vi "Experiment_treatment1_ArtemVer1KG.vi"() -> ()   [LabVIEW 2018]
uses:
  <vilib>/Analysis/1siggen.llb/Ramp Pattern by Samples.vi
  <vilib>/Utility/file.llb/Read From Spreadsheet File (DBL).vi
  <vilib>/Analysis/NI_AALBase.lvlib
  cluster_ip_dll/x64/Release/cluster_ip.dll
panel:
  in  "ratio_perm":dbl=1.0
  in  "length":i32=199847
  out "size(s)":i32[](array[numeric])=[199847, 4]
  out "Working time":dbl=10.736
  in  "Array":string[](array[string])=["Number", "MSE", "Eff. Deg. of Freedom", "Conf. interval size", "Nearest param 1", "Nearest param 2", "Nearest param 3", "Nearest param 4", "Math Exp of param 1", "Math Exp of param 2", "Math Exp of param 3", "Math Exp of param 4", "Stand Dev of param 1", "Stand Dev of param 2", "Stand Dev of param 3", "Stand Dev of param 4", "HPD Intercepts"]
  out "Clusters":i32=2296
  out "Tree built":i32=1
  out "k":dbl=5.363132492919857
  out "Stand Dev":dbl[](array[numeric])=[0.14074417999043268, 0.054181492882835885, 0.0033921981697429128, 12.524756434619329]
  out "Math Exp":dbl[](array[numeric])=[0.6707029123050608, 0.14943200368425694, 1.3769697677746422, 21.22968016405946]
  in  "Database type":u16(ring) items=["Random", "Regular", "Piecewise regular", "DiRect (not realized)"]
  out "MSE":dbl
  out "Nearest Params":sgl[](array[numeric])=[0.68445736, 0.106504805, 1.3702419, 48.924232]
  in  "Load":bool=TRUE
  in  "Params bounds":sgl[][](array[numeric])=[[0.5, 2.12], [0.1, 1.0], [1.37, 1.39], [0.0, 90.0]]
  in  "Database path":path=path "E:/OnEngFiles - science/test labview/4_add_cluster_lib/Plt_200k_h.db"
  in  "Angle bounds":i32[](array[numeric])=[10, 70]
  in  "Path to indicatrices":path=path "E:/OnEngFiles - science/test labview/4_add_cluster_lib/experiment_1000.txt"
  in  "How many to process":u16(ring)=100 items=["All (889)"=889, "100"=100, "300"=300, "1000"=1000]
  in  "Launch":bool=TRUE
  in  "Tab Control":enum32{"Nearest Indicatrix"}(tab)
  out "XY Graph":cluster{"Y":dbl[], "Y":dbl[]}[](graph)=[{"Y"=[10.0, 11.0, 12.0, 13.0, 14.0, 15.0, 16.0, 17.0, 18.0, 19.0, 20.0, 21.0, 22.0, 23.0, 24.0, 25.0, 26.0, 27.0, 28.0, 29.0, 30.0, 31.0, 32.0, 33.0, 34.0, 35.0, 36.0, 37.0, 38.0, 39.0, 40.0, 41.0, 42.0, 43.0, 44.0, 45.0, 46.0, 47.0, 48.0, 49.0, 50.0, 51.0, 52.0, 53.0, 54.0, 55.0, 56.0, 57.0, 58.0, 59.0, 60.0], "Y"=[3.584928234374043e-05, 6.087175402032172e-05, 9.562049901976253e-05, 0.00014104691333700342, 0.00019757729815979622, 0.0002651135616544077, 0.00034308135664397625, 0.0004305081801215161, 0.0005261160539134097, 0.0006284168548823555, 0.0007358019994202503, 0.0008466213987461039, 0.000959249146877231, 0.001072135255465285, 0.0011838439896287526, 0.0012930801075181364, 0.0013987046879531642, 0.0014997423548416817, 0.0015953816629734523, 0.0016849702645666232, 0.0017680062781895245, 0.0018441270646478013, 0.0019130963996333134, 0.0019747908332749266, 0.0020291858490397796, 0.0020763422814356666, 0.0021163933237562708, 0.002149532352204729, 0.0021760017087887502, 0.0021960825196998424, 0.0022100855757161406, 0.0022183432638865374, 0.002221202512987111, 0.002219018696900437, 0.002212150428362565, 0.0022009551689452394, 0.0021857855784477988, 0.002166986527051351, 0.0021448926958249283, 0.0021198266948269017, 0.002092097632614167, 0.00206200007607233, 0.0020298133448228444, 0.001995801089834237, 0.001960211111111111, 0.0019232753743506287, 0.001885210191172391, 0.0018462165319028346, 0.001806480443909125, 0.0017661735521253483, 0.0017254536217018342]}, {"Y"=[10.0, 11.0, 12.0, 13.0, 14.0, 15.0, 16.0, 17.0, 18.0, 19.0, 20.0, 21.0, 22.0, 23.0, 24.0, 25.0, 26.0, 27.0, 28.0, 29.0, 30.0, 31.0, 32.0, 33.0, 34.0, 35.0, 36.0, 37.0, 38.0, 39.0, 40.0, 41.0, 42.0, 43.0, 44.0, 45.0, 46.0, 47.0, 48.0, 49.0, 50.0, 51.0, 52.0, 53.0, 54.0, 55.0, 56.0, 57.0, 58.0, 59.0, 60.0], "Y"=[0.0032144944874749623, 0.0032132298573099827, 0.0029659495363371217, 0.002712444976221678, 0.0026041146328709443, 0.0026259121642624654, 0.002644837766779372, 0.00252843040674818, 0.002242430201747389, 0.0018692780710884763, 0.0015507701572525703, 0.0014033129107546734, 0.0014598002632086123, 0.0016651567756611541, 0.0019170085087040311, 0.0021208737801508017, 0.0022290668182410028, 0.002248300373317722, 0.00222018160530276, 0.00219078906764674, 0.00218647057471567, 0.002205583659012032, 0.0022259928432159367, 0.002220926031811844, 0.00217379465770865, 0.0020852619171353236, 0.001970885484555106, 0.001852323331685977, 0.0017474430288977488, 0.0016641427256584055, 0.0016000347051028934, 0.0015469366635793708, 0.0014969545376869507, 0.0014467263688878807, 0.0013979689937462982, 0.0013547633161661095, 0.0013197453682908813, 0.0012916557375020025, 0.0012655875700386733, 0.0012355249800443844, 0.0011974685704525838, 0.0011512530107925744, 0.0011000865603667544, 0.0010482239528080827, 0.0009982067125814931, 0.0009492368672763391, 0.0008975231352131822, 0.0008383424657175091, 0.0007687260034128252, 0.0006895054184360893, 0.0006059307798655672]}]
  in  "Show graphs":bool
  in  "Calc ME and SD":bool=TRUE
  in  "Clusterization":bool=TRUE
  in  "Use saved tree":bool
  in  "Database path 2":path=path "E:/OnEngFiles - science/test labview/4_add_cluster_lib/complite program/Experiment_treatment1_ArtemVer5_KG02/test_data"
  out "Progress bar":u8(slide)=100 scale=0.0..100.0
  in  "output cluster":T1
  # "Database setup"
  # "Experiment setup"
  # "±"
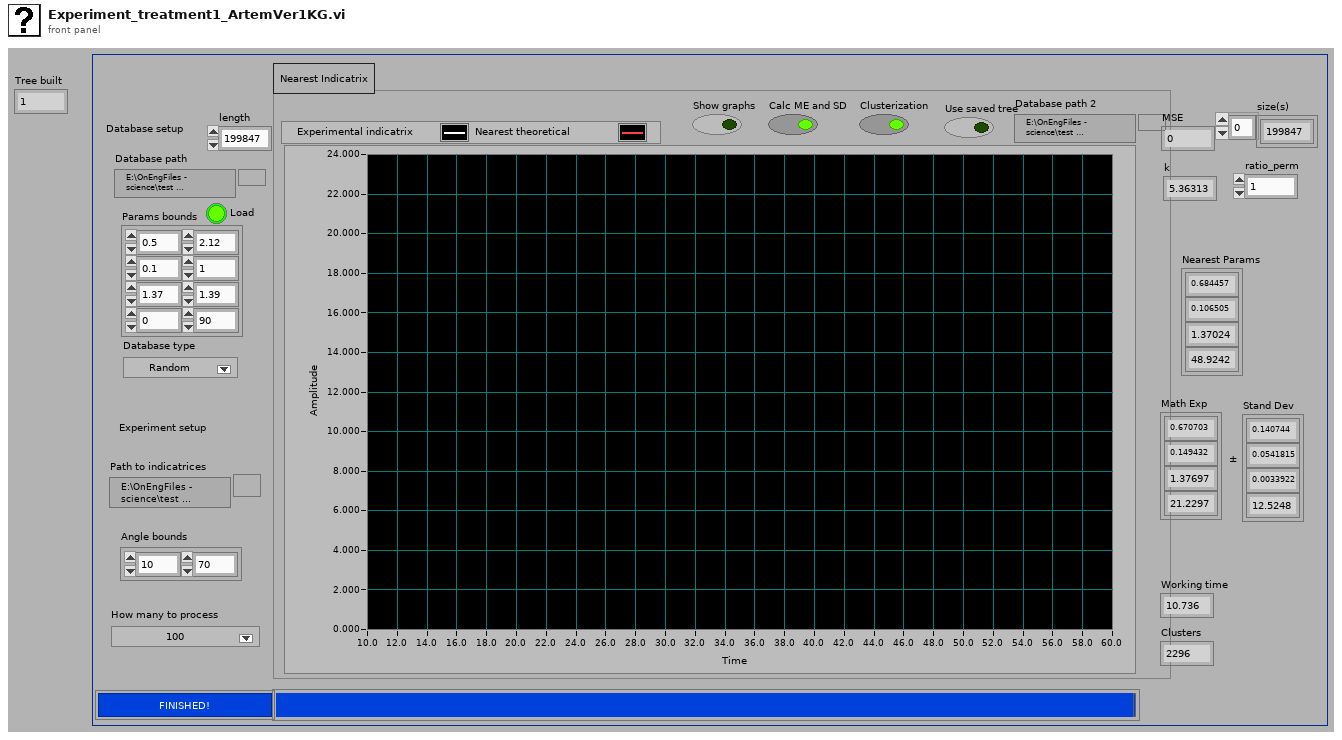
[diagram p1: front panel]
types:
  T1 = cluster{"Angles start":dbl, "Angles end":dbl, "Number of angles":i32, "Params bounds":sgl[][], "Params":sgl[][], "Indicatrices":sgl[][]}
  T2 = typedef "LVStringsAndValuesArrayTypeDef_U16.ctl" = cluster{"String":string, "Value":u16}[]
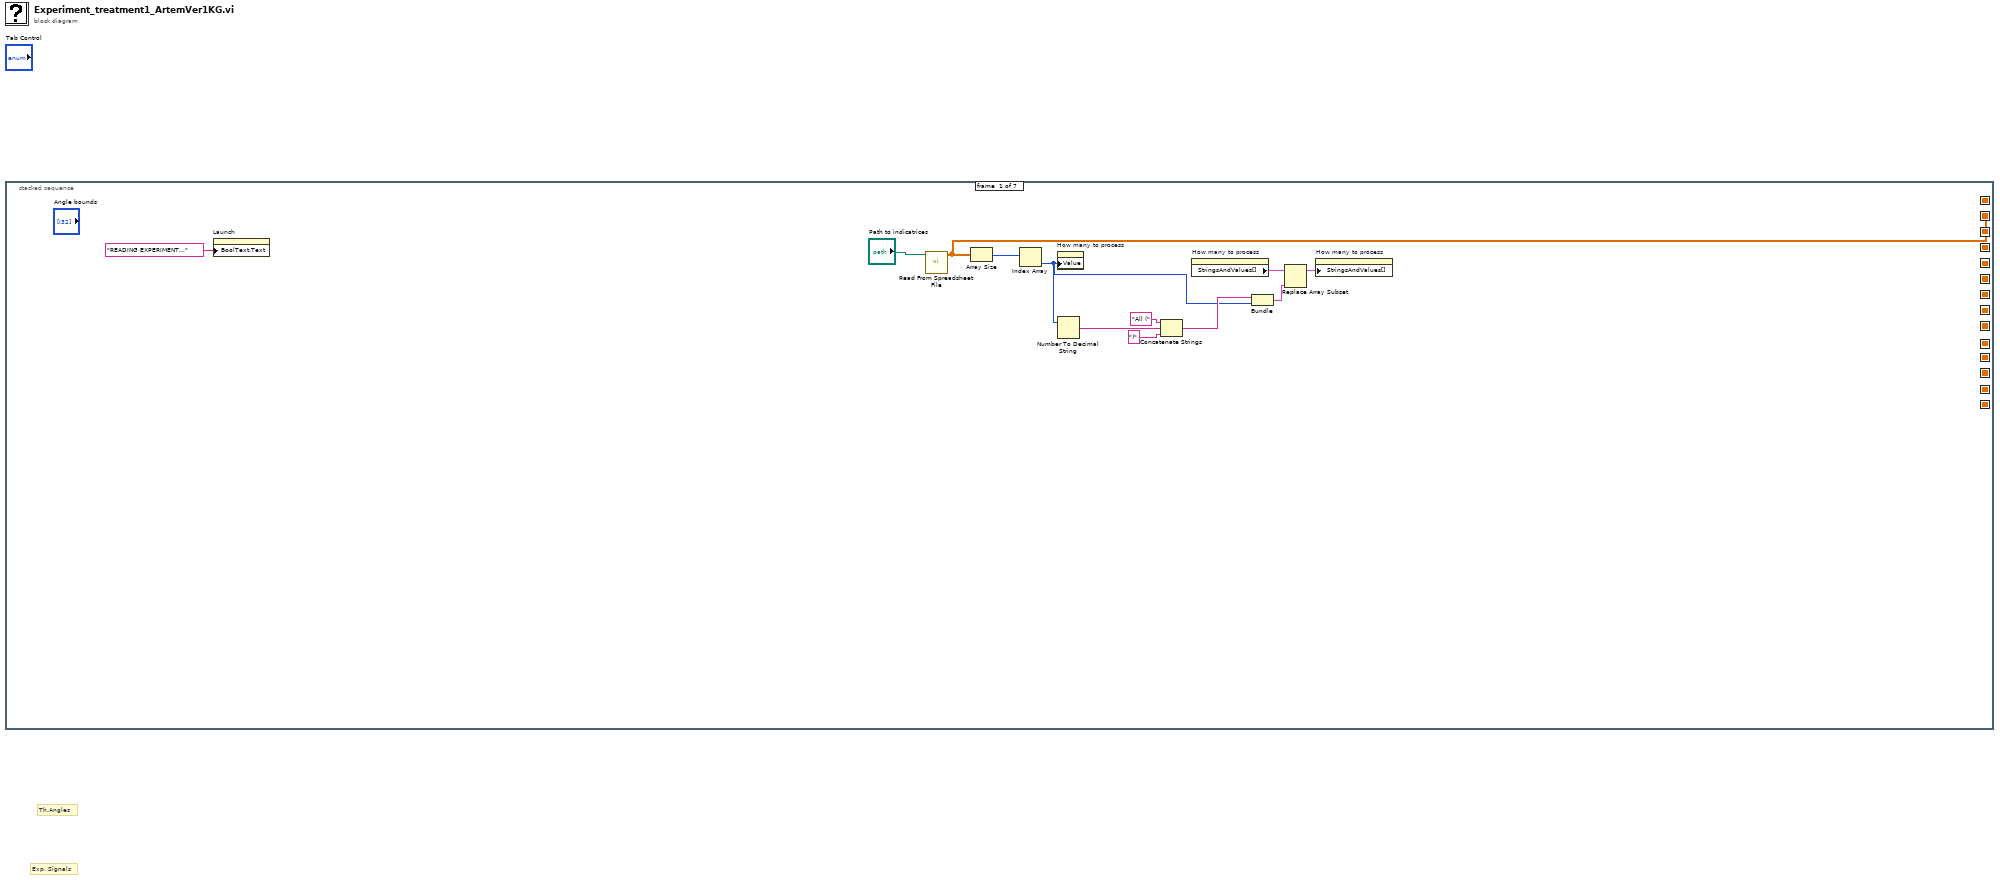
[diagram p0: block diagram]
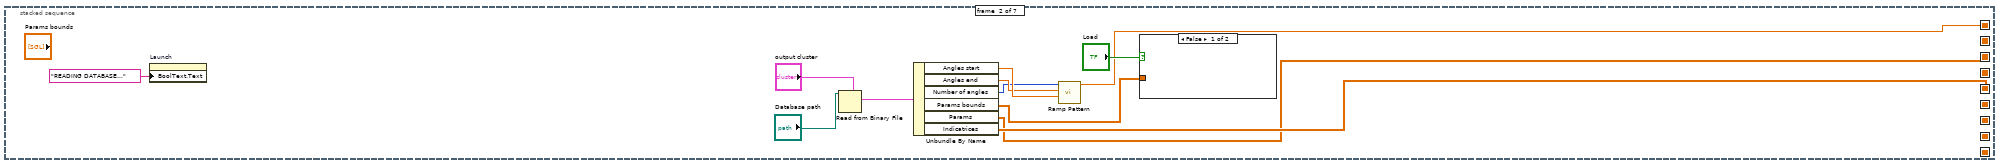
[diagram p2: hidden frame]
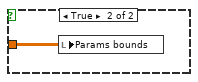
[diagram p3: hidden frame]
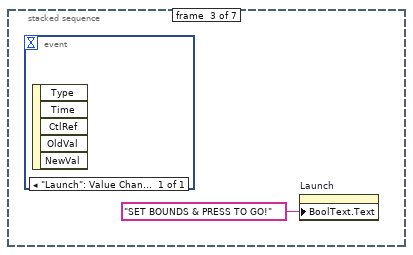
[diagram p4: hidden frame]
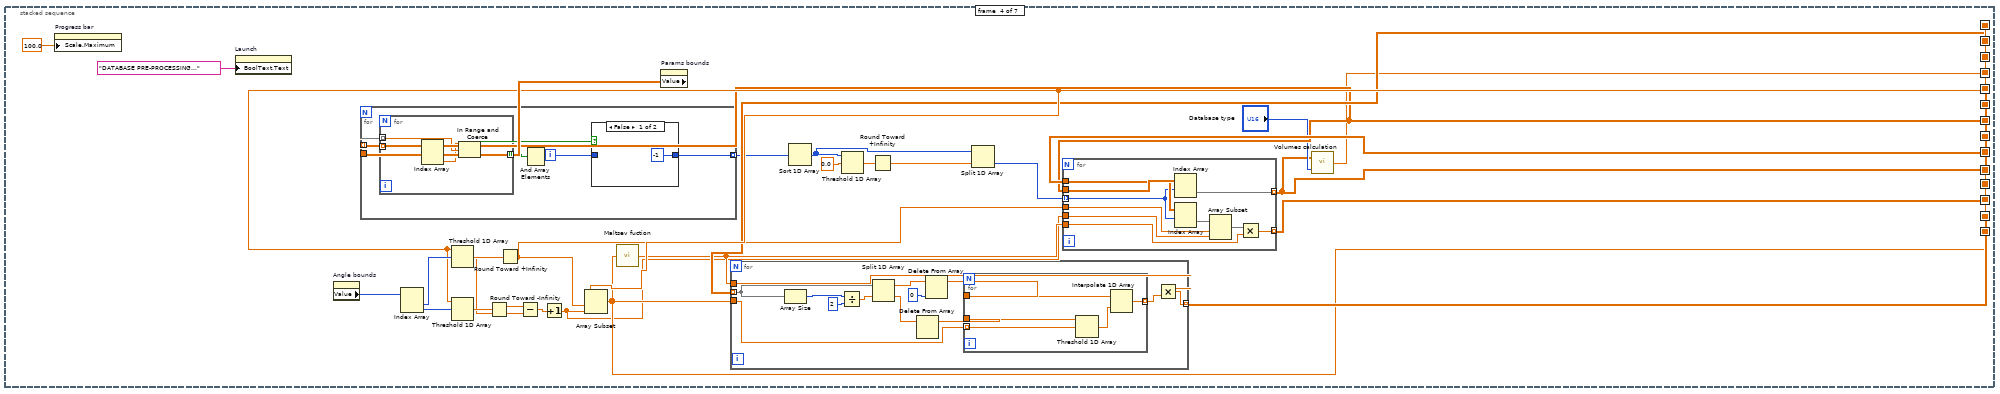
[diagram p5: hidden frame]
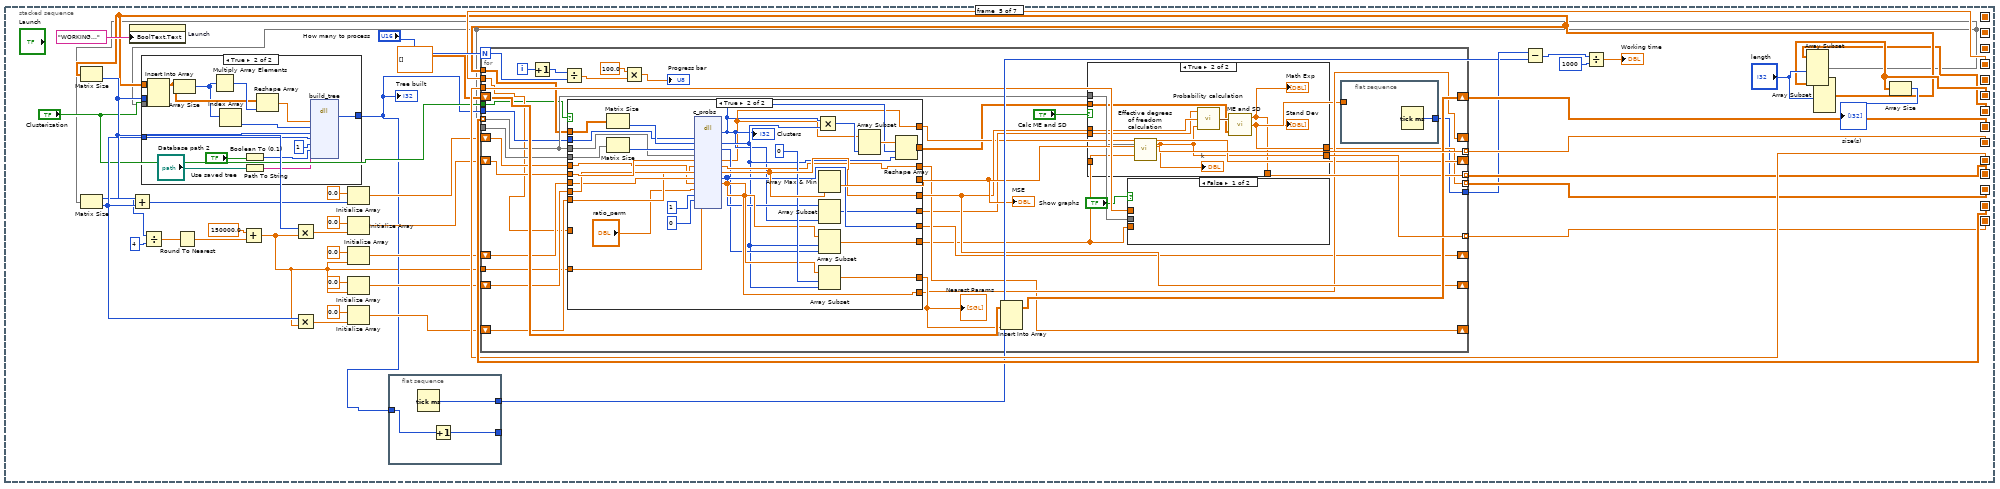
[diagram p7: hidden frame]
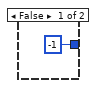
[diagram p8: hidden frame]
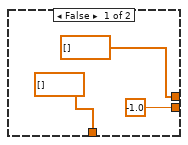
[diagram p9: hidden frame]
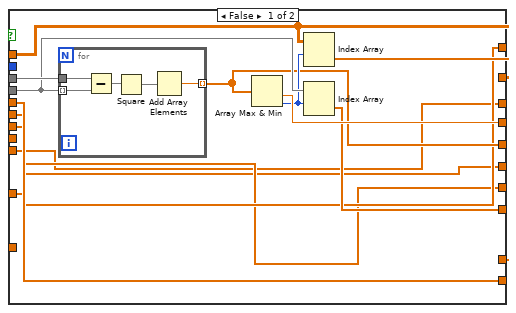
[diagram p10: hidden frame]
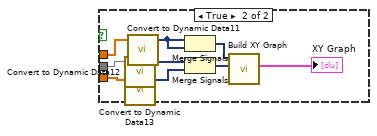
[diagram p11: hidden frame]
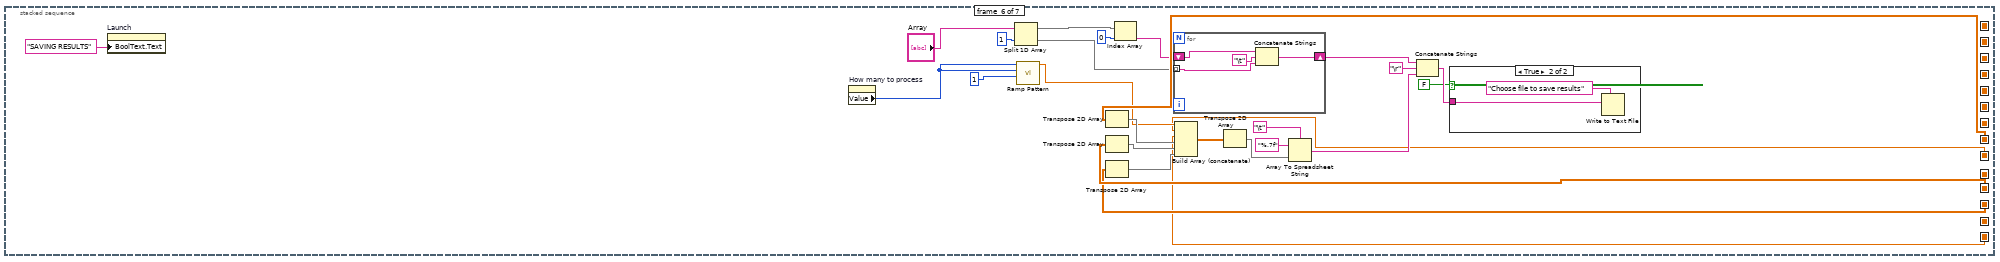
[diagram p12: hidden frame]
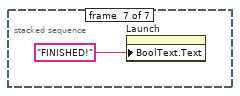
[diagram p14: hidden frame]
diagram:
  # "Th.Angles"
  # "Exp. Signals"
  n1 = stacked-sequence {
    seq-local: [_ w14 _ _ _ _ _] -> [_ _ _ w30 _ _ _]
    seq-local: [_ w21 _ _ _ _ _] -> [_ _ _ w42 _ _ _]
    seq-local: [w1 _ _ _ _ _ _] -> [_ _ _ w45 _ _ _]
    seq-local: [_ w19 _ _ _ _ _] -> [_ _ _ w49 _ _ _]
    seq-local: [_ _ _ w27 _ _ _] -> [_ _ _ _ w101 _ _]
    seq-local: [_ _ _ w41 _ _ _] -> [_ _ _ _ w99 _ _]
    seq-local: [_ _ _ w44 _ _ _] -> [_ _ _ _ w139 _ _]
    seq-local: [_ _ _ w43 _ _ _] -> [_ _ _ _ w138 _ _]
    seq-local: [_ _ _ w29 _ _ _] -> [_ _ _ _ w136 _ _]
    seq-local: [_ _ _ _ w134 _ _] -> [_ _ _ _ _ w293 _]
    seq-local: [_ _ _ _ w135 _ _] -> [_ _ _ _ _ w278 _]
    seq-local: [_ _ _ _ w133 _ _] -> [_ _ _ _ _ w292 _]
    seq-local: [_ _ _ _ w132 _ _] -> [_ _ _ _ _ w291 _]
    seq-local: [_ _ _ _ w131 _ _] -> [_ _ _ _ _ w276 _]
    frame #0 {
      n2 = property on="Launch" class="Bool (strict)"("BoolText.Text"="READING EXPERIMENT..." ("Boolean Text.Text")) -> ()  [unwired: 2 in, 2 out]
      n3 = call-poly <vilib>:"Read From Spreadsheet File.vi"("file path (dialog if empty)"="Path to indicatrices") -> ("all rows"=w1:dbl[][])  [unwired: 6 in, 4 out]
      n4 = Array Size(array=w1) -> (size(s)=w6:i32[])
      n5 = Index Array(array=w6) -> (element=w2:i32)  [unwired: 1 in]
      n6 = property on="How many to process" class="Ring (strict)"("Value"=w2) -> ()  [unwired: 2 in, 2 out]
      n7 = Number To Decimal String(number=w2) -> (decimal integer string=w3:string)  [unwired: 1 in]
      n8 = Concatenate Strings("All (" ("String"), w3, ")" ("String")) -> (w5:string)
      n9 = property on="How many to process" class="Ring (strict)"() -> ("StringsAndValues[]"=w10:T2)  [unwired: 2 in, 2 out]
      n10 = Bundle(w5, w2) -> (w8:cluster{string, i32})  [unwired: 1 in]
      n11 = Replace Array Subset(array=w10, new element=w8) -> (w11:T2)  [unwired: 1 in]
      n12 = property on="How many to process" class="Ring (strict)"("StringsAndValues[]"=w11) -> ()  [unwired: 2 in, 2 out]
    }
    frame #1 {
      n13 = property on="Launch" class="Bool (strict)"("BoolText.Text"="READING DATABASE..." ("Boolean Text.Text")) -> ()  [unwired: 2 in, 2 out]
      n14 = Read from Binary File(5:"output cluster", 11:"Database path") -> (2:w24:T1)  [unwired: 4 in, 3 out]
      n15 = Unbundle By Name(w24) -> ("Angles start"=w20:dbl, "Angles end"=w18:dbl, "Number of angles"=w17:i32, "Params bounds"=w16:sgl[][], "Params"=w14:sgl[][], "Indicatrices"=w21:sgl[][])
      n16 = call-poly <vilib>:"Ramp Pattern.vi"("start"=w20, "end"=w18, "samples"=w17) -> ("Ramp Pattern"=w19:dbl[])  [unwired: 7 in, 1 out]
      n17 = case shown="False" "Load" {
        tunnel: w16 -> [_ w25]
        frame False {
        }
        frame True {
          n18 = local write "Params bounds"(w25) -> ()
        }
      }
    }
    frame #2 {
      n19 = event shown="[0] \"Launch\": Value Change" {
        selector: _ -> [_]
        dyn-events: _ -> [_]
        timeout: _ -> [_]
        event "Launch": Value Change {
          n20 = event-data() -> ()  [unwired: 1 in, 5 out]
        }
      }
      n21 = property on="Launch" class="Bool (strict)"("BoolText.Text"="SET BOUNDS & PRESS TO GO!" ("Boolean Text.Text")) -> ()  [unwired: 2 in, 2 out]
    }
    frame #3 {
      n22 = property on="Progress bar" class="Slide (strict)"("Scale.Maximum"=100.0 ("Scale.Range:Maximum")) -> ()  [unwired: 2 in, 2 out]
      n23 = property on="Launch" class="Bool (strict)"("BoolText.Text"="DATABASE PRE-PROCESSING..." ("Boolean Text.Text")) -> ()  [unwired: 2 in, 2 out]
      n24 = property on="Angle bounds" class="Arr (strict)"() -> ("Value"=w53:i32[])  [unwired: 2 in, 2 out]
      n25 = Index Array(array=w53) -> (element #1=w52:i32, element #2=w46:i32)  [unwired: 2 in]
      n26 = Threshold 1D Array(2:w52, 3:w49) -> (0:w51:dbl)  [unwired: 1 in]
      n27 = Threshold 1D Array(2:w46, 3:w49) -> (0:w50:dbl)  [unwired: 1 in]
      n28 = Round Toward -Infinity(1:w50) -> (0:w48:dbl)
      n29 = Round Toward +Infinity(x=w51) -> (ceil(x): smallest int >= x=w38:dbl)
      n30 = Subtract(x=w48, y=w38) -> (x-y=w47:dbl)
      n31 = Increment(x=w47) -> (x+1=w39:dbl)
      n32 = Array Subset(array=w49, index=w38, length=w39) -> (w43:dbl[])
      n33 = call "Maltsev fuction.vi"("Angles"=w43) -> ("Maltsev fuction"=w40:dbl[])
      n34 = property on="Params bounds" class="Arr (strict)"() -> ("Value"=w54:sgl[][])  [unwired: 2 in, 2 out]
      n35 = for {
        tunnel: w30 -> [w87] mode=indexing
        tunnel: w54 -> [w89]
        tunnel: [w84] -> w37 mode=indexing
        i -> [w85]
        n36 = for {
          tunnel: w89 -> [w96] mode=indexing
          tunnel: w87 -> [w95] mode=indexing
          tunnel: [w92] -> w88 mode=indexing
          n37 = Index Array(array=w96) -> (element #1=w94:sgl, element #2=w93:sgl)  [unwired: 2 in]
          n38 = In Range and Coerce(upper limit=w93, x=w95, lower limit=w94) -> (In Range?=w92:bool)  [unwired: 1 out]
        }
        n39 = And Array Elements(Boolean array=w88) -> (logical AND=w86:bool)
        n40 = case shown="False" w86 {
          tunnel: w85 -> [_ w91]
          tunnel: [-1 w91] -> w84
          frame False {
          }
          frame True {
          }
        }
      }
      n41 = for {
        tunnel: w45 -> [w72] mode=indexing
        tunnel: w43 -> [w69]
        tunnel: w40 -> [w68]
        tunnel: [w66] -> w44 mode=indexing
        n42 = Array Size(array=w72) -> (size(s)=w76:i32)
        n43 = Divide(x=w76, y=2) -> (x/y=w75:dbl)
        n44 = Split 1D Array(array=w72, index=w75) -> (first subarray=w78:dbl[], second subarray=w77:dbl[])
        n45 = Delete From Array(array=w77) -> (array with subset deleted=w70:dbl[])  [unwired: 2 in, 1 out]
        n46 = Delete From Array(array=w78, index=0) -> (array with subset deleted=w71:dbl[])  [unwired: 1 in, 1 out]
        n47 = for {
          tunnel: w71 -> [w82]
          tunnel: w70 -> [w81]
          tunnel: w69 -> [w80] mode=indexing
          tunnel: [w79] -> w67 mode=indexing
          n48 = Threshold 1D Array(2:w80, 3:w81) -> (0:w83:dbl)  [unwired: 1 in]
          n49 = Interpolate 1D Array(1:w83, 2:w82) -> (0:w79:dbl)
        }
        n50 = Multiply(x=w68, y=w67) -> (x*y=w66:dbl[])
      }
      n51 = Sort 1D Array(array=w37) -> (sorted array=w33:i32[])
      n52 = Threshold 1D Array(2:0.0 ("threshold y"), 3:w33) -> (0:w35:dbl)  [unwired: 1 in]
      n53 = Round Toward +Infinity(x=w35) -> (ceil(x): smallest int >= x=w34:dbl)
      n54 = Split 1D Array(array=w33, index=w34) -> (second subarray=w32:i32[])  [unwired: 1 out]
      n55 = for {
        tunnel: w30 -> [w65]
        tunnel: w42 -> [w64]
        tunnel: [w63] -> w27 mode=indexing
        tunnel: [w60] -> w41 mode=indexing
        tunnel: w40 -> [w59]
        tunnel: w39 -> [w58]
        tunnel: w38 -> [w57]
        tunnel: w32 -> [w56] mode=indexing
        n56 = Index Array(array=w65, index (row)=w56) -> (element=w63:sgl[])  [unwired: 1 in]
        n57 = Index Array(array=w64, index (row)=w56) -> (element=w61:sgl[])  [unwired: 1 in]
        n58 = Array Subset(array=w61, index=w57, length=w58) -> (w62:sgl[])
        n59 = Multiply(x=w62, y=w59) -> (x*y=w60:dbl[])
      }
      n60 = call "Volumes calculation.vi"("Ring"="Database type", "Params"=w27) -> ("Volumes"=w29:sgl[])
    }
    frame #4 {
      n61 = property on="Launch" class="Bool (strict)"("BoolText.Text"="WORKING..." ("Boolean Text.Text")) -> ()  [unwired: 2 in, 2 out]
      n62 = flat-sequence {
        tunnel: [w144] -> w109
        tunnel: w104 -> [w143]
        tunnel: [w142] -> _
        frame #0 {
          n63 = Tick Count (ms)() -> (millisecond timer value=w144:u32)
          n64 = Increment(x=w143) -> (x+1=w142:i32)
        }
      }
      n65 = Array Subset(array=w99, length (row)="length") -> (w98:dbl[][])  [unwired: 3 in]
      n66 = Matrix Size(0:w98) -> (1:w114:i32, 2:w117:i32)
      n67 = Divide(x=w114, y=4) -> (x/y=w112:dbl)
      n68 = Round To Nearest(number=w112) -> (nearest integer value=w111:dbl)
      n69 = Add(x=150000.0 ("element"), y=w111) -> (x+y=w97:dbl)
      n70 = Multiply(x=w117, y=w97) -> (x*y=w118:dbl)
      n71 = Initialize Array(0.0 ("element"), w97) -> (w121:dbl[])
      n72 = Initialize Array(0.0 ("element"), w97) -> (w122:dbl[])
      n73 = Initialize Array(0.0 ("element"), w118) -> (w116:dbl[])
      n74 = Array Subset(array=w101, length (row)="length") -> (w100:sgl[][])  [unwired: 3 in]
      n75 = Matrix Size(0:w100) -> (2:w130:i32)  [unwired: 1 out]
      n76 = Add(x=w130, y=w117) -> (x+y=w129:i32)
      n77 = case shown="True" "Clusterization" {
        tunnel: w130 -> [_ w160]
        tunnel: w100 -> [_ w153]
        tunnel: w98 -> [_ w152]
        tunnel: [-1 ("return type") w151] -> w104
        tunnel: w117 -> [_ w150]
        frame False {
        }
        frame True {
          n78 = Insert Into Array(array=w153, index (col)=w160, new element=w152) -> (w155:sgl[][])  [unwired: 1 in]
          n79 = Array Size(array=w155) -> (size(s)=w154:i32[])
          n80 = Multiply Array Elements(1:w154) -> (0:w156:i32)
          n81 = Index Array(array=w154) -> (element=w158:i32)  [unwired: 1 in]
          n82 = Path To String(path="Database path 2") -> (string=w146:string)
          n83 = Boolean To (0,1)(Boolean="Use saved tree") -> (0, 1=w148:i16)
          n84 = Reshape Array(w155, w156) -> (w157:sgl[])
          n85 = dll-call lib="E:/OnEngFiles - science/test labview/4_add_cluster_lib/git_version/Cluster_IP/actual_code/cluster_ip_dll/x64/Release/cluster_ip.dll" fn="build_tree"("data"=w157, "number_points"=w158, "hiden_size"=w160, "mesured_size"=w150, "save"=1, "use_saved"=w148, "folder_name"=w146) -> ("return type"=w151:i32)  [unwired: 10 in, 2 out]
        }
      }
      "Tree built" <- w104
      n86 = Multiply(x=w130, y=w97) -> (x*y=w128:dbl)
      n87 = Initialize Array(0.0 ("element"), w129) -> (w120:dbl[])
      n88 = Initialize Array(0.0 ("element"), w128) -> (w123:dbl[])
      n89 = for {
        N: "How many to process" -> [w195]
        tunnel: w100 -> [w176]
        tunnel: w98 -> [w175]
        tunnel: w139 -> [w185] mode=indexing
        tunnel: w138 -> [w191]
        shift-right: [w187] -> w134
        shift-left: sgl[][] [] ("Params") -> [w188]
        tunnel: w136 -> [w164]
        tunnel: [w190] -> w135 mode=indexing
        tunnel: [w186] -> w133 mode=indexing
        tunnel: [w168] -> w132 mode=indexing
        tunnel: [w189] -> w131 mode=indexing
        shift-right: [w170] -> _
        shift-left: w123 -> [w183]
        shift-right: [w181] -> _
        shift-left: w122 -> [w165]
        shift-right: [w174] -> _
        shift-left: w121 -> [w182]
        shift-right: [w178] -> _
        shift-left: w120 -> [w184]
        tunnel: w104 -> [w180]
        shift-right: [w177] -> _
        shift-left: w116 -> [w166]
        tunnel: [w167] -> w110
        tunnel: "Clusterization" -> [w163]
        tunnel: w97 -> [w161]
        i -> [w196]
        n90 = Increment(x=w196) -> (x+1=w192:i32)
        n91 = Divide(x=w192, y=w195) -> (x/y=w197:dbl)
        n92 = case shown="True" w163 {
          tunnel: [w222 w259] -> w190
          tunnel: w185 -> [w223 w254]
          tunnel: w184 -> [w215 w231]
          tunnel: w183 -> [w214 w253]
          tunnel: w165 -> [_ w252]
          tunnel: w182 -> [w213 w251]
          tunnel: [w217 w250] -> w181
          tunnel: w180 -> [_ w249]
          tunnel: [w221 w247] -> w179
          tunnel: [w215 w246] -> w178
          tunnel: w166 -> [w212 w245]
          tunnel: [w214 w232] -> w170
          tunnel: [w212 w244] -> w177
          tunnel: w176 -> [w216 w243]
          tunnel: w175 -> [w220 w242]
          tunnel: [w213 w241] -> w174
          tunnel: [w211 w240] -> w173
          tunnel: [w218 w238] -> w171
          tunnel: [w216 w233] -> w169
          tunnel: w164 -> [w211 _]
          tunnel: w161 -> [_ w229]
          frame False {
            n93 = for {
              tunnel: w223 -> [w228]
              tunnel: w220 -> [w227] mode=indexing
              tunnel: [w225] -> w217 mode=indexing
              n94 = Subtract(x=w228, y=w227) -> (x-y=w224:dbl[])
              n95 = Square(x=w224) -> (x^2=w226:dbl[])
              n96 = Add Array Elements(numeric array=w226) -> (sum=w225:dbl)
            }
            n97 = Array Max & Min(array=w217) -> (min value=w222:dbl, min index (indices)=w219:i32)  [unwired: 2 out]
            n98 = Index Array(array=w216, index (row)=w219) -> (element=w221:sgl[])  [unwired: 1 in]
            n99 = Index Array(array=w220, index (row)=w219) -> (element=w218:dbl[])  [unwired: 1 in]
          }
          frame True {
            n100 = Matrix Size(0:w243) -> (2:w258:i32)  [unwired: 1 out]
            n101 = Matrix Size(0:w242) -> (2:w257:i32)  [unwired: 1 out]
            n102 = dll-call lib="E:/OnEngFiles - science/test labview/4_add_cluster_lib/git_version/Cluster_IP/actual_code/cluster_ip_dll/x64/Release/cluster_ip.dll" fn="c_probs"("number_points"=w249, "hiden_size"=w258, "mesured_size"=w257, "measure"=w254, "centers"=w253, "indicatrix"=w245, "dist_s"=w252, "weights"=w251, "closest"=w231, "ratio_perm"="ratio_perm", "is_build_tree"=1, "load"=i8 0, "max_clust_num"=w229) -> ("return type"=w234:i32, "hiden_size"=w235:i32, "mesured_size"=w239:i32, "centers"=w232:dbl[], "indicatrix"=w244:dbl[], "dist_s"=w250:dbl[], "weights"=w241:i32[], "closest"=w246:dbl[])  [unwired: 9 in, 2 out]
            "Clusters" <- w234
            n103 = Multiply(x=w234, y=w235) -> (x*y=w237:i32)
            n104 = Array Max & Min(array=w250) -> (min value=w259:dbl)  [unwired: 3 out]
            n105 = Array Subset(array=w241, length=w234) -> (w240:i32[])  [unwired: 1 in]
            n106 = Array Subset(array=w246, index=w235, length=w239) -> (w238:dbl[])
            n107 = Array Subset(array=w246, index=0, length=w235) -> (w247:dbl[])
            n108 = Array Subset(array=w232, length=w237) -> (w236:dbl[])  [unwired: 1 in]
            n109 = Reshape Array(w236, w234, w235) -> (w233:dbl[][])
          }
        }
        "Nearest Params" <- w179
        "MSE" <- w190
        n110 = Multiply(x=100.0, y=w197) -> (x*y=→"Progress bar":dbl)
        n111 = Insert Into Array(array=w188, new element=w179) -> (w187:sgl[][])  [unwired: 2 in]
        n112 = case shown="True" "Calc ME and SD" {
          tunnel: [-1.0 ("effective degrees of freedom") w208] -> w189
          tunnel: [dbl[] [] ("ME") w207] -> w186
          tunnel: w185 -> [_ w206]
          tunnel: w181 -> [_ w205]
          tunnel: w173 -> [_ w204]
          tunnel: w171 -> [_ w203]
          tunnel: w169 -> [_ w202]
          tunnel: [dbl[] [] ("SD") w201] -> w168
          frame False {
          }
          frame True {
            n113 = call "Effective degrees of freedom calculation.vi"("nearest theoretical function from database"=w203, "experimental function"=w206) -> ("effective degrees of freedom"=w208:dbl)  [unwired: 1 out]
            "k" <- w208
            n114 = call "Probability calculation.vi"("effective degrees of freedom"=w208, "MSE array"=w205, "Volumes"=w204) -> ("Sorted Probabilities"=w209:cluster{dbl, dbl, i32}[])
            n115 = call "ME and SD.vi"("Array"=w202, "Sorted Probabilities"=w209) -> ("SD"=w201:dbl[], "ME"=w207:dbl[])  [unwired: 1 in]
            "Math Exp" <- w207
            "Stand Dev" <- w201
          }
        }
        n116 = case shown="False" "Show graphs" {
          tunnel: w191 -> [_ w262]
          tunnel: w185 -> [_ w263]
          tunnel: w171 -> [_ w261]
          frame False {
          }
          frame True {
            n117 = call "Convert to Dynamic Data12"("Array"=w263) -> ("Dynamic Data Type"=w266:dynamicdata)  [unwired: 3 in]
            n118 = call "Convert to Dynamic Data13"("Array"=w261) -> ("Dynamic Data Type"=w260:dynamicdata)  [unwired: 3 in]
            n119 = call "Convert to Dynamic Data11"("Array"=w262) -> ("Dynamic Data Type"=w264:dynamicdata)  [unwired: 3 in]
            n120 = Merge Signals(w264, w264) -> (w265:dynamicdata)
            n121 = Merge Signals(w266, w260) -> (w267:dynamicdata)
            n122 = call "Build XY Graph"("Y Input"=w267, "X Input"=w265) -> ("XY Graph"=→"XY Graph":cluster{"Y":dbl[], "Y":dbl[]}[])  [unwired: 8 in, 1 out]
          }
        }
        n123 = flat-sequence {
          tunnel: w168 -> [_]
          tunnel: [w210] -> w167
          frame #0 {
            n124 = Tick Count (ms)() -> (millisecond timer value=w210:u32)
          }
        }
      }
      n125 = Subtract(x=w110, y=w109) -> (x-y=w107:u32)
      n126 = Divide(x=w107, y=u32 1000) -> (x/y=→"Working time":dbl)
      n127 = Array Size(array=w101) -> (size(s)=→"size(s)":i32[])
    }
    frame #5 {
      n128 = property on="Launch" class="Bool (strict)"("BoolText.Text"="SAVING RESULTS" ("Boolean Text.Text")) -> ()  [unwired: 2 in, 2 out]
      n129 = property on="How many to process" class="Ring (strict)"() -> ("Value"=w290:u16)  [unwired: 2 in, 2 out]
      n130 = Split 1D Array(array="Array", index=1) -> (first subarray=w272:string[], second subarray=w273:string[])
      n131 = call-poly <vilib>:"Ramp Pattern.vi"("start"=1, "end"=w290, "samples"=w290) -> ("Ramp Pattern"=w279:dbl[])  [unwired: 7 in, 1 out]
      n132 = Transpose 2D Array(2D array=w293) -> (transposed array=w289:sgl[][])
      n133 = Transpose 2D Array(2D array=w292) -> (transposed array=w288:dbl[][])
      n134 = Transpose 2D Array(2D array=w291) -> (transposed array=w287:dbl[][])
      n135 = Index Array(array=w272, index=0) -> (element=w270:string)
      n136 = for {
        tunnel: w273 -> [w299] mode=indexing
        shift-right: [w298] -> w277
        shift-left: w270 -> [w301]
        n137 = Concatenate Strings(w301, "\t", w299) -> (w298:string)
      }
      n138 = Build Array (concatenate)(w279, w278, w276, w289, w288, w287) -> (w284:dbl[][])
      n139 = Transpose 2D Array(2D array=w284) -> (transposed array=w283:dbl[][])
      n140 = Array To Spreadsheet String(delimiter (Tab)="\t", array=w283, 3:"%.7f" ("format (%.3f)")) -> (spreadsheet string=w286:string)
      n141 = Concatenate Strings(w277, "\r", w286) -> (w285:string)
      n142 = case shown="True" FALSE {
        tunnel: w285 -> [_ w297]
        frame False {
        }
        frame True {
          n143 = Write to Text File(prompt (Choose or enter file path)="Choose file to save results", text=w297) -> ()  [unwired: 2 in, 3 out]
        }
      }
    }
    frame #6 {
      n144 = property on="Launch" class="Bool (strict)"("BoolText.Text"="FINISHED!" ("Boolean Text.Text")) -> ()  [unwired: 2 in, 2 out]
    }
  }
